vi "FileRead_CalConst.vi"(8 "error in":errorcluster, 11 "file path (use dialog)":path=path "") -> (0 "error out":errorcluster, 2 "Calibration Constants":T1(array[cluster]) {"PSlope" format="%#.13f"; "NSlope" format="%#.13f"; "AvgSlope" format="%#.13f"; "Center" format="%#.13f"; "Offset" format="%#.13f"})   [LabVIEW 2015]
uses:
  <vilib>/Utility/file.llb/Read Delimited Spreadsheet (DBL).vi
panel:
  # "x1"
  # "x10"
  # "x100"
  # "x1000"
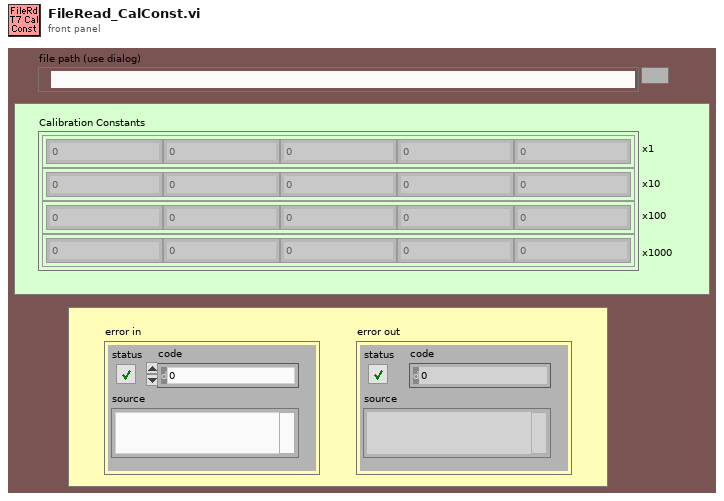
[diagram p1: front panel]
types:
  T1 = cluster{"PSlope":dbl, "NSlope":dbl, "AvgSlope":dbl, "Center":dbl, "Offset":dbl}[]
  T2 = cluster{"Numeric":dbl, "Numeric":dbl, "Numeric":dbl, "Numeric":dbl, "Numeric":dbl}[]
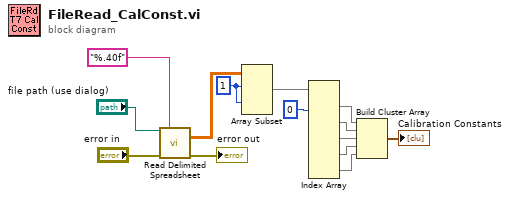
[diagram p0: block diagram]
diagram:
  w12 = 1 ("index")
  n1 = call-poly <vilib>:"Read Delimited Spreadsheet.vi"("file path (dialog if empty)"="file path (use dialog)", "format (%.3f)"="%.40f", "error in (no error)"="error in") -> ("all rows"=w13:dbl[][], "error out"=→"error out":errorcluster)  [unwired: 7 in, 4 out]
  n2 = Array Subset(array=w13, index (row)=w12, index (col)=w12) -> (w11:dbl[][])  [unwired: 2 in]
  n3 = Index Array(array=w11, index (col) #1=0 ("index (row)")) -> (element #1=w10:dbl[], element #2=w9:dbl[], element #3=w8:dbl[], element #4=w7:dbl[], element #5=w6:dbl[])  [unwired: 9 in]
  n4 = Build Cluster Array(w10, w9, w8, w7, w6) -> (→"Calibration Constants":T2)
